vi "Load Teams.vi"() -> (2 "Names":string[](array[string]), 3 "Available Teams":refnum<class "Team.lvclass">[](array[class]))   [LabVIEW 2020, in "SB App.lvlib" / "SB App.lvclass"]
uses:
  SB App.lvclass
  SquareBattle/Team/Team.lvclass
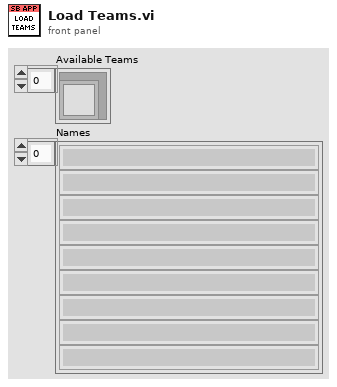
[diagram p1: front panel]
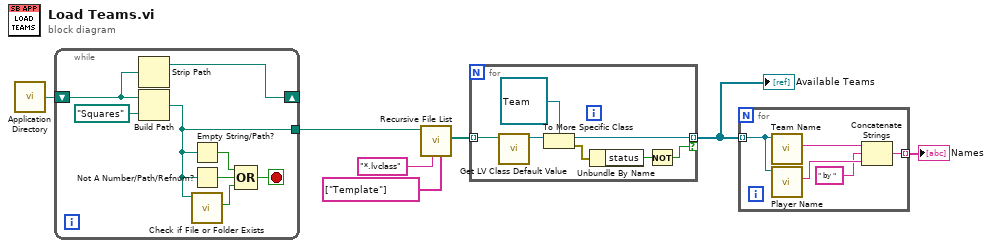
[diagram p0: block diagram]
diagram:
  n1 = call <vilib>:"Application Directory.vi"() -> ("Application Directory"=w7:path)
  n2 = while {
    shift-right: [w13] -> _
    shift-left: w7 -> [w14]
    tunnel: [w12] -> w1
    stop <- w8 stop-if-true
    n3 = Strip Path(path=w14) -> (stripped path=w13:path)  [unwired: 1 out]
    n4 = Build Path(base path=w14, name or relative path=path "Squares") -> (appended path=w12:path)
    n5 = Empty String/Path?(string/path=w12) -> (empty?=w10:bool)
    n6 = Not A Number/Path/Refnum?(number/path/refnum=w12) -> (NaN/Path/Refnum?=w11:bool)
    n7 = call <vilib>:"Check if File or Folder Exists.vi"("path"=w12) -> ("file or folder exists?"=w9:bool)  [unwired: 8 in, 2 out]
    n8 = Compound Arithmetic op=OR(w10, w11, w9) -> (w8:bool)
  }
  n9 = call <vilib>:"Recursive File List.vi"("Folders to Exclude"=string[] ["Template"], "pattern"="*.lvclass", "Folder Path"=w1) -> ("All Files in Dir"=w4:path[])  [unwired: 4 in, 4 out]
  n10 = for {
    tunnel: w4 -> [w22] mode=indexing
    tunnel: [w19] -> w3 mode=indexing if=w16
    n11 = call <vilib>:"Get LV Class Default Value.vi"("class path"=w22) -> ("object"=w21:refnum<class>)  [unwired: 9 in, 1 out]
    n12 = To More Specific Class(target class=refnum<class "Team.lvclass"> refnum ("SquareBattle:Team"), reference=w21) -> (specific class reference=w19:refnum<class "Team.lvclass">, error out=w18:errorcluster)  [unwired: 1 in]
    n13 = Unbundle By Name(w18) -> ("status"=w17:bool)
    n14 = Not(x=w17) -> (.not. x?=w16:bool)
  }
  "Available Teams" <- w3
  n15 = for {
    tunnel: w3 -> [w27] mode=indexing
    tunnel: [w23] -> w2 mode=indexing
    n16 = call-dynamic "Team Name.vi"("Team in"=w27) -> ("Team Name"=w26:string)  [unwired: 10 in]
    n17 = call-dynamic "Player Name.vi"("Team"=w27) -> ("Player Name"=w25:string)  [unwired: 10 in]
    n18 = Concatenate Strings(w26, " by " ("string"), w25) -> (w23:string)
  }
  "Names" <- w2
